vi "TDMS_Viewer.vi"(11 "Data Directory":path=path "C:/Users/LAV-UFSC-2023/Documents/LAV-TCC/Dados-Experimentos/Dados-Bancada-LABVIEW") -> ()   [LabVIEW 2022 SP3]
uses:
  <vilib>/Utility/TDMS File Viewer/NI_TDMS File Viewer.lvlib
panel:
  in  "Python Script Path":path=path "C:/Users/LAV-UFSC-2023/Documents/LAV-TCC/PyScript/readTDMS.py" caption="Python Module Path"
  out "error out":errorcluster
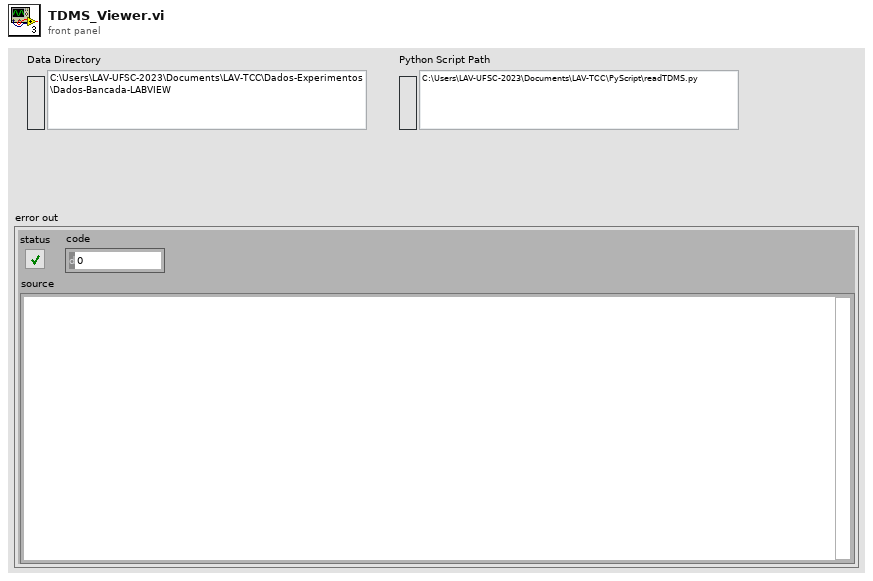
[diagram p1: front panel]
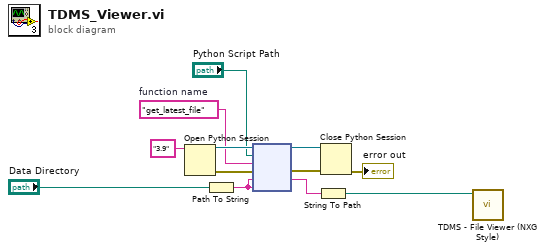
[diagram p0: block diagram]
diagram:
  w11 = "get_latest_file"  # function name
  n1 = Open Python Session(python version="3.9" ("Python version")) -> (session out=w12:refnum<k35>, error out=w10:errorcluster)  [unwired: 2 in]
  n2 = Path To String(path="Data Directory") -> (string=w4:string)
  n3 = node(w12, "Python Script Path", w11, w10, w4, w4) -> (w6:refnum<k35>, w5:errorcluster, w8:string)  [unwired: 1 in, 2 out]
  n4 = String To Path(string=w8) -> (path=w9:path)
  n5 = Close Python Session(session in=w6, error in=w5) -> (11:→"error out":errorcluster)
  n6 = call <vilib>:"TDMS - File Viewer (NXG Style).vi"("file in"=w9) -> ()  [unwired: 9 in, 2 out]
